vi "Get LVObject.vi"(8 "error in (no error)":errorcluster, 9 "Object Type":refnum<class>, 10 "Offset":i32, 11 "JSON String containing Flattened Object":string) -> (0 "error out":errorcluster, 1 "Object out":refnum<class>)   [LabVIEW 2015, in "JSONtext.lvlib"]
doc: "Gets LabVIEW Object that has been flattened and stored as a JSON String."
uses:
  JSONtext.lvlib
  Advance past String.vi
  String Subset.vi
  support/Strip Quotes and Unescape.vi
  support/Unescape JSON string.vi
  Parsing Error.vi
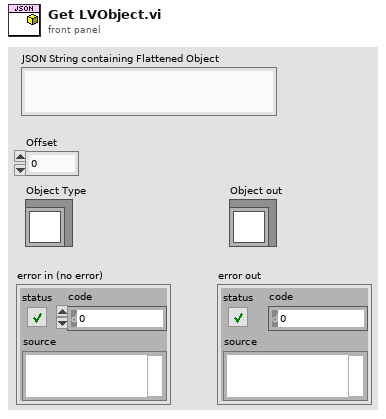
[diagram p1: front panel]
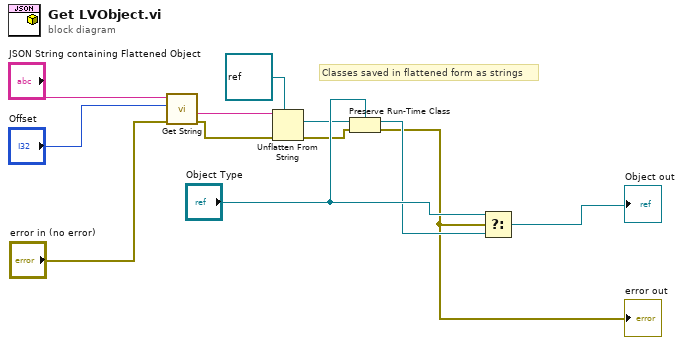
[diagram p0: block diagram]
diagram:
  # "Classes saved in flattened form as strings"
  n1 = call "Get String.vi"("error in (no error)"="error in (no error)", "Offset"="Offset", "JSON"="JSON String containing Flattened Object") -> ("error out"=w11:errorcluster, "String"=w4:string)  [unwired: 6 in, 1 out]
  n2 = Unflatten From String(type=refnum<class> refnum ("LabVIEW Object"), binary string=w4, error in (no error)=w11) -> (value=w5:refnum<class>, error out=w6:errorcluster)  [unwired: 2 in, 1 out]
  n3 = Preserve Run-Time Class(object in=w5, error in=w6, 2:"Object Type") -> (object out=w8:refnum<class>, error out=w7:errorcluster)
  "error out" <- w7
  n4 = Select(t="Object Type", s=w7, f=w8) -> (s? t:f=→"Object out":refnum<class>)
